vi "Sistema de Vacio 2.0.vi"() -> ()   [LabVIEW 2019]
uses:
  PortConfig.ctl
  <vilib>/Instr/_visa.llb/VISA Configure Serial Port (Instr).vi
panel:
  in  "System OFF":bool
  out "IG Filament Status 2":string
  out "VAC/ATM":bool caption="Boolean"
  out "TP AV/NAV":bool caption="Boolean"
  out "BP AV/NAV":bool caption="Boolean"
  in  "Ion Gauge":bool
  out "IG AV/NAV 2":bool caption="Boolean"
  in  "Turbo Pump":bool
  in  "System ON":bool
  in  "Backing Pump":bool
  in  "Disconnect":bool
  out "IG AV/NAV":bool caption="Boolean"
  out "Ion Gauge Controller":errorcluster
  out "Vacuum Controller":errorcluster
  out "Branking":bool
  out "Stopped":bool
  out "Starting Delay":bool
  out "Accelerating":bool
  out "Stopping Normal Delay":bool
  out "Fault Branking":bool
  out "Stopping Short Delay":bool
  out "Running":bool
  out "Backing Pump":bool
  out "Turbo Normal Speed":bool
  out "Turbo Power [W]":dbl(knob) scale=0.0..110.0
  out "Turbo Power [W]":dbl
  out "Turbo Speed":dbl(knob) scale=0.0..100.0
  out "Turbo Speed":dbl
  out "Vent Valve":bool
  out "PS Temp":dbl
  out "Internal Temp":dbl
  out "Apagado":bool
  out "B_Online":bool caption="Boolean"
  out "IG_Online":bool caption="Boolean"
  out "IG [TORR]":string
  out "IG3":dbl(knob) scale=1e-09..1e-07 scale format="%#_3e"
  out "IG":dbl(knob) scale=1e-09..0.001 scale format="%#_6e"
  out "IG1":dbl(knob) scale=1e-05..0.001 scale format="%#_3e"
  out "IG2":dbl(knob) scale=1e-07..1e-05 scale format="%#_3e"
  out "CG2 [TORR]":string
  out "CG2L":dbl(knob) scale=0.01..800.0
  out "CG2":dbl(knob) scale=0.0..800.0
  out "CG1 [TORR]":string
  out "CG1L":dbl(knob) scale=0.01..800.0
  out "CG1":dbl(knob) scale=0.0..800.0
  out "IG Filament Status":string
  out "Activo":bool
  out "ActivoIG":bool caption="Activo"
  out "Emission Current Status":string
  out "IG Code\nIG code":string
  out "IG Status":string
  out "Software Version":string
  out "Serial Number ; PIC Version":string
  out "Software Version":string
  out "TIC Model":string
  in  "Ion Gauge":refnum<visa-resource-name>="COM12"
  in  "Bombas":refnum<visa-resource-name>="COM16"
  in  "?":bool
  in  "Error In":errorcluster
  # "CONTROLS CONNECTION"
  # "VACUUM SYSTEM CONTROL"
  # "Error Handling"
  # "IG CONTROL"
  # "CONTROLLER"
  # "TURBO-PUMP DATA"
  # "TURBO-PUMP STATUS"
  # "PUMP STATUS"
  # "CONTROLLER"
  # "CONVECTRON DATA"
  # "ION GAUGE DATA"
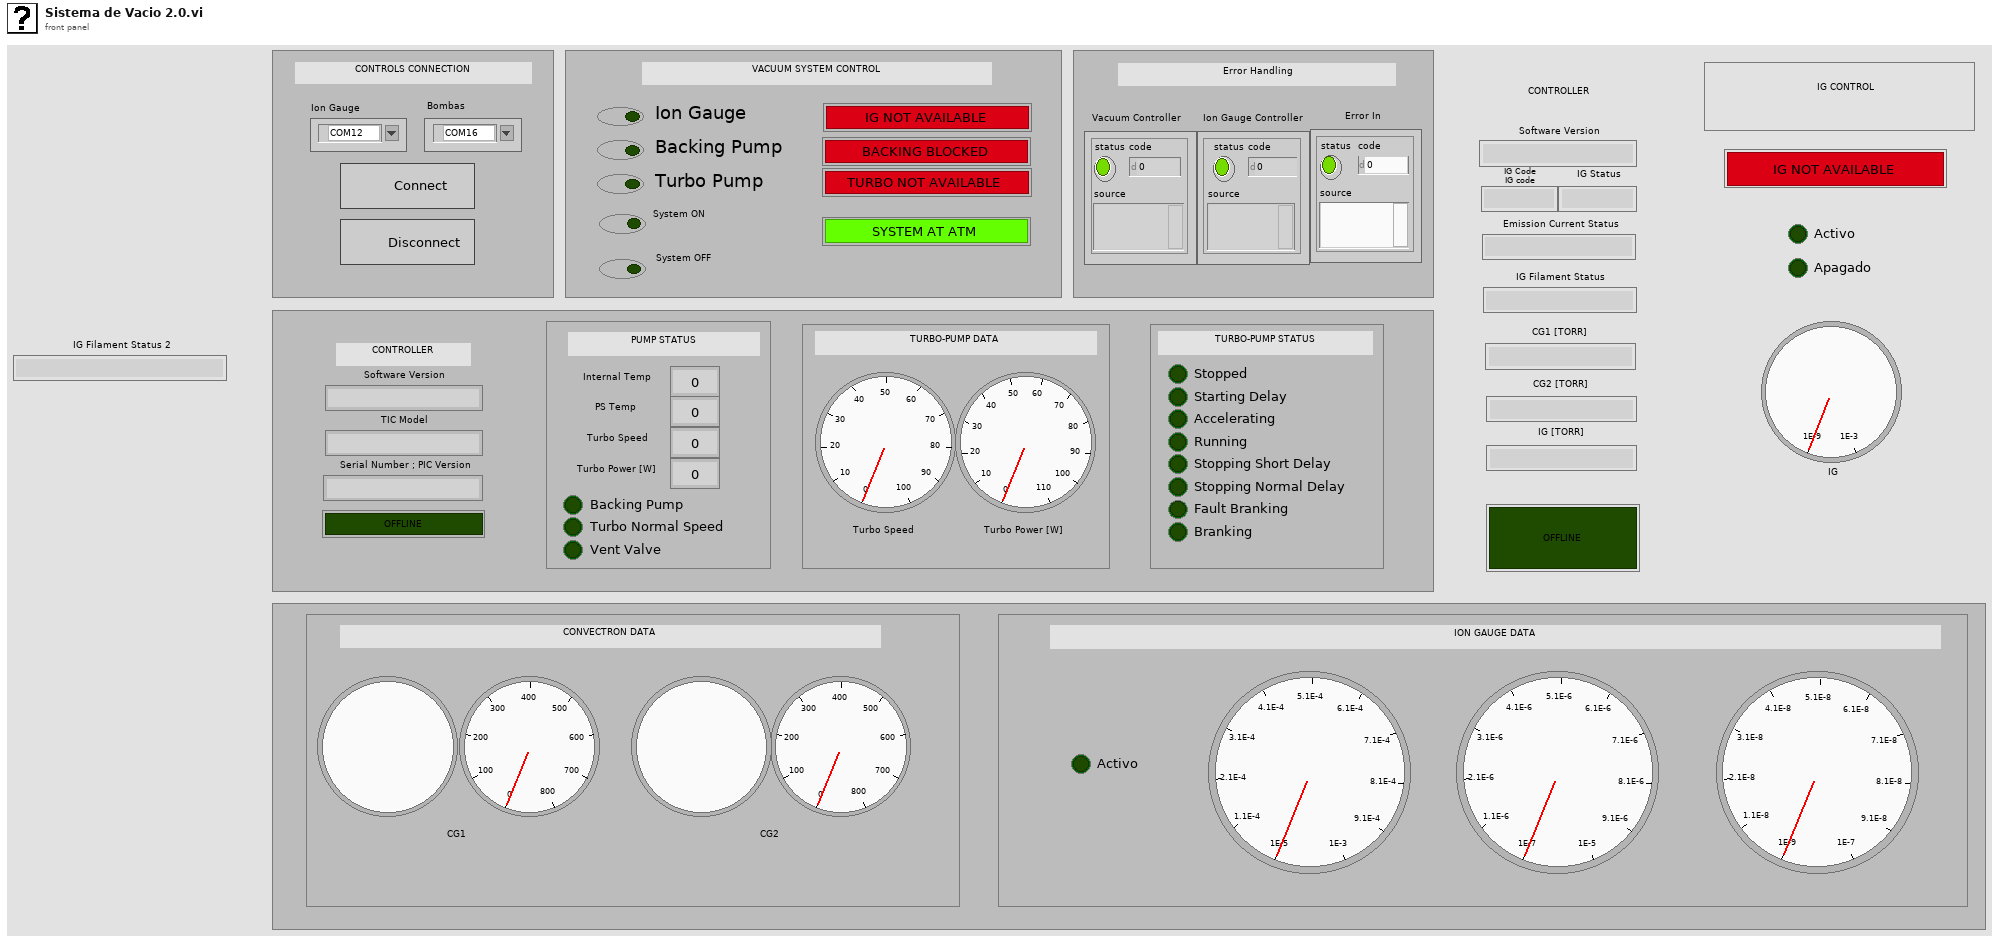
[diagram p1: front panel]
types:
  T1 = typedef "PortConfig.ctl" = cluster{"baud rate":u32, "data bits":u16, "parity":enum16{"None", "Odd", "Even", "Mark", "Space"}, "stop bits":u16}
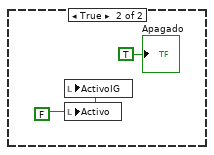
[diagram p2: hidden frame]
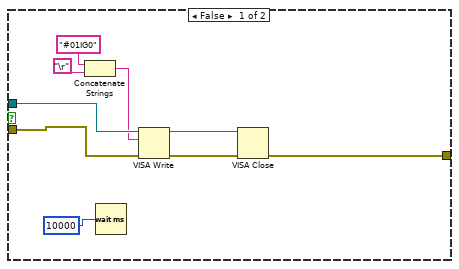
[diagram p3: hidden frame]
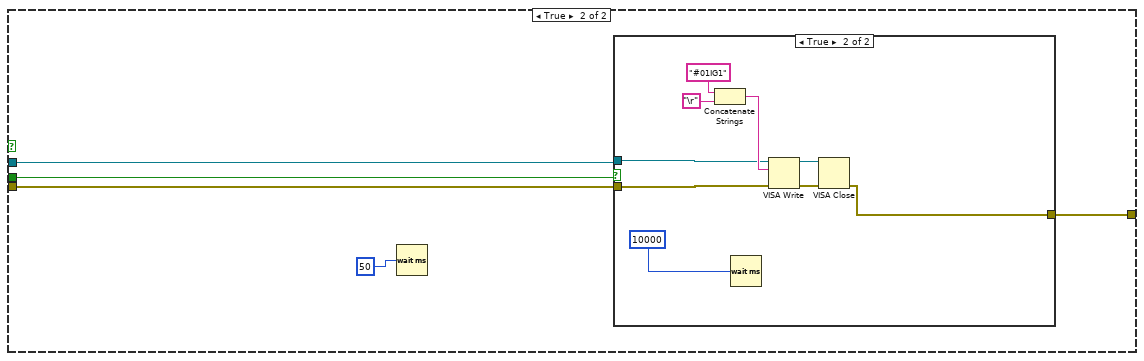
[diagram p4: hidden frame]
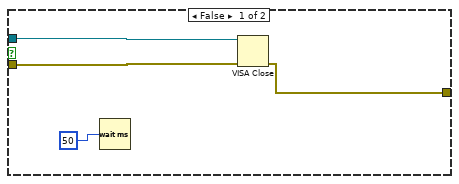
[diagram p5: hidden frame]
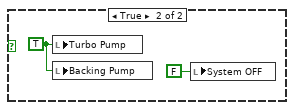
[diagram p7: hidden frame]
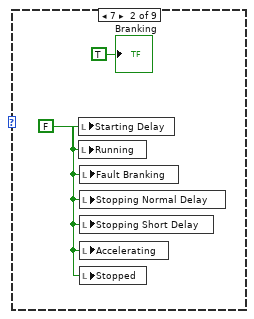
[diagram p11: hidden frame]
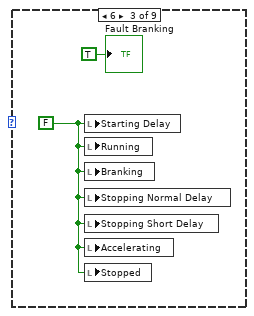
[diagram p12: hidden frame]
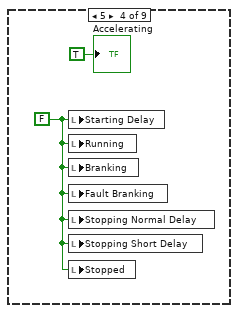
[diagram p13: hidden frame]
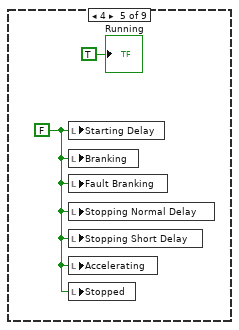
[diagram p14: hidden frame]
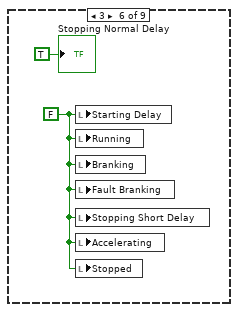
[diagram p15: hidden frame]
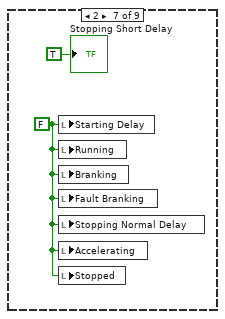
[diagram p16: hidden frame]
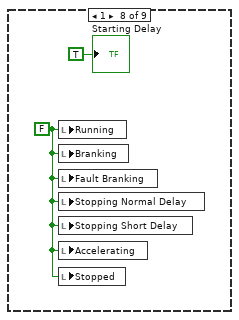
[diagram p17: hidden frame]
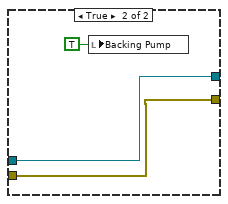
[diagram p19: hidden frame]
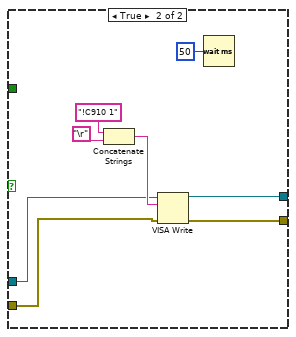
[diagram p20: hidden frame]
diagram:
  n1 = while {
    tunnel: "Error In" -> [w33]
    tunnel: [w33] -> w21
    stop <- "?" stop-if-true
    w22 = FALSE ("IG AV/NAV 2")
    w23 = " " ("CG1 [TORR]")
    w24 = 0.0 ("IG2")
    w25 = FALSE ("Apagado")
    w26 = FALSE ("Turbo Pump")
    w27 = FALSE ("Running")
    w29 = 0.0 ("Turbo Speed")
    w28 = FALSE ("IG_Online")
    w30 = " " ("TIC Model")
    n2 = local write "TP AV/NAV"(w27) -> ()
    n3 = local write "BP AV/NAV"(w27) -> ()
    n4 = local write "Running"(w27) -> ()
    n5 = local write "Branking"(w27) -> ()
    n6 = local write "Fault Branking"(w27) -> ()
    n7 = local write "Accelerating"(w27) -> ()
    n8 = local write "Stopping Normal Delay"(w27) -> ()
    n9 = local write "Stopping Short Delay"(w27) -> ()
    n10 = local write "Starting Delay"(w27) -> ()
    n11 = local write "Stopped"(w27) -> ()
    n12 = local write "VAC/ATM"(w27) -> ()
    n13 = local write "IG AV/NAV 2"(w27) -> ()
    n14 = local write "IG2"(w24) -> ()
    n15 = local write "IG1"(w24) -> ()
    n16 = local write "IG"(w24) -> ()
    n17 = local write "CG1"(w24) -> ()
    n18 = local write "CG1L"(w24) -> ()
    n19 = local write "IG3"(w24) -> ()
    n20 = local write "Apagado"(w25) -> ()
    n21 = local write "IG_Online"(w25) -> ()
    n22 = local write "ActivoIG"(w25) -> ()
    n23 = local write "Activo"(w25) -> ()
    n24 = local write "System ON"(w26) -> ()
    n25 = local write "Turbo Pump"(w26) -> ()
    n26 = local write "Backing Pump"(w26) -> ()
    n27 = local write "Ion Gauge"(w26) -> ()
    n28 = local write "IG AV/NAV 2"(w22) -> ()
    n29 = local write "IG AV/NAV"(w22) -> ()
    n30 = local write "System OFF"(w22) -> ()
    n31 = local write "CG1 [TORR]"(w23) -> ()
    n32 = local write "CG2 [TORR]"(w23) -> ()
    n33 = local write "IG [TORR]"(w23) -> ()
    n34 = local write "IG Filament Status"(w23) -> ()
    n35 = local write "Emission Current Status"(w23) -> ()
    n36 = local write "Software Version"(w23) -> ()
    n37 = local write "IG Code\nIG code"(w23) -> ()
    n38 = local write "IG Status"(w23) -> ()
    n39 = local write "Turbo Speed"(w29) -> ()
    n40 = local write "Turbo Speed"(w29) -> ()
    n41 = local write "Turbo Power [W]"(w29) -> ()
    n42 = local write "Turbo Power [W]"(w29) -> ()
    n43 = local write "Internal Temp"(w29) -> ()
    n44 = local write "PS Temp"(w29) -> ()
    n45 = local write "TIC Model"(w30) -> ()
    n46 = local write "Software Version"(w30) -> ()
    n47 = local write "Serial Number ; PIC Version"(w30) -> ()
    n48 = local write "IG_Online"(w28) -> ()
    n49 = local write "B_Online"(w28) -> ()
    n50 = local write "Vent Valve"(w28) -> ()
    n51 = local write "Turbo Normal Speed"(w28) -> ()
    n52 = local write "Backing Pump"(w28) -> ()
    n53 = Wait (ms)(milliseconds to wait=u32 200) -> ()  [unwired: 1 out]
  }
  n54 = flat-sequence {
    tunnel: w21 -> [w52]
    tunnel: [w52] -> w14
    tunnel: [w37] -> w13
    tunnel: [w36] -> w12
    tunnel: [w35] -> w11
    tunnel: [w34] -> w10
    tunnel: [w113] -> w9
    tunnel: w14 -> [w113]
    tunnel: w13 -> [w98]
    tunnel: w12 -> [w97]
    tunnel: w11 -> [w80]
    tunnel: w10 -> [w79]
    tunnel: [w78] -> w8
    tunnel: [w77] -> w7
    tunnel: [w59] -> w6
    tunnel: [w58] -> w5
    tunnel: [w53] -> w2
    tunnel: [w55] -> w1
    tunnel: [w120] -> w15
    tunnel: [w121] -> w16
    tunnel: [w122] -> w17
    tunnel: [w123] -> w18
    tunnel: [w124] -> w19
    tunnel: w9 -> [w124]
    tunnel: w8 -> [w119]
    tunnel: w7 -> [w118]
    tunnel: w6 -> [w117]
    tunnel: w5 -> [w116]
    tunnel: [w114] -> w4
    tunnel: [w115] -> w3
    tunnel: w2 -> [w115]
    tunnel: w1 -> [w114]
    frame #0 {
      n55 = Unbundle By Name(T1 {"baud rate"=9600, "data bits"=8, "parity"=enum."None", "stop bits"=10} ("Serial Settings")) -> ("data bits"=w48:u16, "parity"=w47:enum16{"None", "Odd", "Even", "Mark", "Space"}, "stop bits"=w49:u16)  [unwired: 1 out]
      n56 = Unbundle By Name(T1 {"baud rate"=9600, "data bits"=8, "parity"=enum."None", "stop bits"=10} ("Serial Settings")) -> ("data bits"=w43:u16, "parity"=w42:enum16{"None", "Odd", "Even", "Mark", "Space"}, "stop bits"=w44:u16)  [unwired: 1 out]
      n57 = call-poly "VISA Configure Serial Port"("VISA resource name"="Bombas", "data bits (8)"=w48, "parity (0:none)"=w47, "stop bits (10: 1 bit)"=w49) -> ("VISA resource name out"=w39:refnum<visa-resource-name>, "error out"=w38:errorcluster)  [unwired: 10 in]
      n58 = call-poly "VISA Configure Serial Port"("VISA resource name"="Ion Gauge", "data bits (8)"=w43, "parity (0:none)"=w42, "stop bits (10: 1 bit)"=w44) -> ("VISA resource name out"=w41:refnum<visa-resource-name>, "error out"=w40:errorcluster)  [unwired: 10 in]
      n59 = VISA Flush I/O Buffer(VISA resource name=w39, error in (no error)=w38) -> (VISA resource name out=w37:refnum<visa-resource-name>, error out=w36:errorcluster)  [unwired: 1 in]
      n60 = VISA Flush I/O Buffer(VISA resource name=w41, error in (no error)=w40) -> (VISA resource name out=w35:refnum<visa-resource-name>, error out=w34:errorcluster)  [unwired: 1 in]
    }
    frame #1 {
      n61 = Concatenate Strings("?V910", "\r") -> (w110:string)
      n62 = Concatenate Strings("#01IGS", "\r") -> (w90:string)
      n63 = VISA Write(VISA resource name=w98, write buffer=w110, error in (no error)=w97) -> (VISA resource name out=w109:refnum<visa-resource-name>, error out=w108:errorcluster)  [unwired: 1 out]
      n64 = VISA Write(VISA resource name=w80, write buffer=w90, error in (no error)=w79) -> (VISA resource name out=w94:refnum<visa-resource-name>, error out=w95:errorcluster)  [unwired: 1 out]
      n65 = VISA Read(VISA resource name=w109, byte count=u32 10, error in (no error)=w108) -> (VISA resource name out=w100:refnum<visa-resource-name>, read buffer=w105:string, error out=w99:errorcluster)  [unwired: 1 out]
      n66 = VISA Read(VISA resource name=w94, byte count=13, error in (no error)=w95) -> (VISA resource name out=w78:refnum<visa-resource-name>, read buffer=w96:string, error out=w77:errorcluster)  [unwired: 1 out]
      n67 = Search/Split String(string=w105, search string/char (-)=" ") -> (match + rest of string=w103:string)  [unwired: 1 in, 2 out]
      n68 = Search/Split String(string=w96, search string/char (-)="IG ", offset (0)=3) -> (match + rest of string=w81:string)  [unwired: 2 out]
      "IG Filament Status 2" <- w81
      n69 = Search/Split String(string=w103, search string/char (-)=";") -> (substring before match=w102:string)  [unwired: 1 in, 2 out]
      n70 = Equal?(x=" 0", y=w102) -> (x = y?=w54:bool)
      n71 = Not(x=w54) -> (.not. x?=w53:bool)
      n72 = Search/Split String(string=w81, search string/char (-)="O", offset (0)=3) -> (match + rest of string=w82:string)  [unwired: 2 out]
      n73 = VISA Flush I/O Buffer(VISA resource name=w100, error in (no error)=w99) -> (VISA resource name out=w61:refnum<visa-resource-name>, error out=w60:errorcluster)  [unwired: 1 in]
      n74 = local write "Backing Pump"(w53) -> ()
      n75 = Concatenate Strings("?V907", "\r") -> (w71:string)
      n76 = Concatenate Strings("OFF", "\r") -> (w83:string)
      n77 = VISA Write(VISA resource name=w61, write buffer=w71, error in (no error)=w60) -> (VISA resource name out=w70:refnum<visa-resource-name>, error out=w69:errorcluster)  [unwired: 1 out]
      n78 = Equal?(x=w83, y=w82) -> (x = y?=w57:bool)
      n79 = Not(x=w57) -> (.not. x?=w56:bool)
      n80 = VISA Read(VISA resource name=w70, byte count=u32 10, error in (no error)=w69) -> (VISA resource name out=w75:refnum<visa-resource-name>, read buffer=w66:string, error out=w76:errorcluster)  [unwired: 1 out]
      n81 = local write "Ion Gauge"(w56) -> ()
      n82 = Search/Split String(string=w66, search string/char (-)=" ") -> (match + rest of string=w64:string)  [unwired: 1 in, 2 out]
      n83 = VISA Flush I/O Buffer(VISA resource name=w75, error in (no error)=w76) -> (VISA resource name out=w59:refnum<visa-resource-name>, error out=w58:errorcluster)  [unwired: 1 in]
      n84 = Search/Split String(string=w64, search string/char (-)=";") -> (substring before match=w63:string)  [unwired: 1 in, 2 out]
      n85 = Equal?(x=" 0", y=w63) -> (x = y?=w74:bool)
      n86 = Not(x=w74) -> (.not. x?=w55:bool)
      n87 = local write "Turbo Pump"(w55) -> ()
    }
    frame #2 {
      n88 = VISA Flush I/O Buffer(VISA resource name=w117, error in (no error)=w116) -> (VISA resource name out=w121:refnum<visa-resource-name>, error out=w120:errorcluster)  [unwired: 1 in]
      n89 = VISA Flush I/O Buffer(VISA resource name=w119, error in (no error)=w118) -> (VISA resource name out=w123:refnum<visa-resource-name>, error out=w122:errorcluster)  [unwired: 1 in]
    }
  }
  n90 = while {
    tunnel: w19 -> [_]
    tunnel: w18 -> [w245]
    tunnel: w17 -> [w244]
    tunnel: w16 -> [w243]
    tunnel: w15 -> [w242]
    shift-right: [w138] -> _
    shift-left: w3 -> [w184]
    shift-right: [w137] -> _
    shift-left: w4 -> [w185]
    stop <- "Disconnect" stop-if-true
    n91 = flat-sequence {
      tunnel: w242 -> [w464]
      tunnel: w243 -> [w465]
      tunnel: [w465] -> w187
      tunnel: [w464] -> w186
      tunnel: w185 -> [w459]
      tunnel: w184 -> [w463]
      tunnel: [w462] -> w145
      tunnel: [w461] -> w144
      tunnel: ["Backing Pump"] -> w143
      tunnel: ["Turbo Pump"] -> w142
      tunnel: [w471] -> w240
      tunnel: [w470] -> w239
      tunnel: w187 -> [w491]
      tunnel: w186 -> [w490]
      tunnel: [w469] -> w150
      tunnel: [w468] -> w148
      tunnel: [w467] -> w147
      tunnel: [w466] -> w146
      tunnel: w145 -> [w467]
      tunnel: w144 -> [w468]
      tunnel: w143 -> [w466]
      tunnel: w142 -> [w469]
      tunnel: w240 -> [w506]
      tunnel: w239 -> [w512]
      tunnel: [w503] -> w238
      tunnel: [w502] -> w237
      tunnel: [w500] -> w157
      tunnel: [w499] -> w154
      tunnel: [w498] -> w151
      tunnel: w150 -> [w497]
      tunnel: [w497] -> w149
      tunnel: w148 -> [w498]
      tunnel: w147 -> [w500]
      tunnel: w146 -> [w499]
      tunnel: w238 -> [w527]
      tunnel: w237 -> [w526]
      tunnel: [w523] -> w236
      tunnel: [w522] -> w235
      tunnel: [w521] -> w163
      tunnel: [w520] -> w158
      tunnel: w157 -> [w519]
      tunnel: [w519] -> w156
      tunnel: w154 -> [w518]
      tunnel: [w518] -> w153
      tunnel: w151 -> [w521]
      tunnel: w149 -> [w520]
      tunnel: w236 -> [w554]
      tunnel: w235 -> [w553]
      tunnel: [w546] -> w234
      tunnel: [w545] -> w233
      tunnel: w163 -> [w542]
      tunnel: [w542] -> w162
      tunnel: [w541] -> w160
      tunnel: w158 -> [w541]
      tunnel: w156 -> [w540]
      tunnel: [w540] -> w155
      tunnel: w153 -> [w539]
      tunnel: [w539] -> w152
      tunnel: w234 -> [w578]
      tunnel: w233 -> [w577]
      tunnel: [w570] -> w232
      tunnel: [w569] -> w231
      tunnel: [w565] -> w169
      tunnel: [w564] -> w166
      tunnel: w162 -> [w563]
      tunnel: [w563] -> w161
      tunnel: w160 -> [w562]
      tunnel: [w562] -> w159
      tunnel: w155 -> [w565]
      tunnel: w152 -> [w564]
      tunnel: [w561] -> w135
      tunnel: w232 -> [w594]
      tunnel: w231 -> [w593]
      tunnel: [w592] -> w230
      tunnel: [w591] -> w229
      tunnel: [w590] -> w175
      tunnel: [w589] -> w172
      tunnel: w169 -> [w588]
      tunnel: [w588] -> w168
      tunnel: w166 -> [w587]
      tunnel: [w587] -> w165
      tunnel: w161 -> [w590]
      tunnel: w159 -> [w589]
      tunnel: [w586] -> w136
      tunnel: w135 -> [w586]
      tunnel: [w585] -> w131
      tunnel: w130 -> [w585]
      tunnel: w230 -> [w621]
      tunnel: w229 -> [w620]
      tunnel: [w616] -> w228
      tunnel: [w615] -> w227
      tunnel: w175 -> [w613]
      tunnel: [w613] -> w174
      tunnel: w172 -> [w612]
      tunnel: [w612] -> w171
      tunnel: w168 -> [w611]
      tunnel: [w611] -> w167
      tunnel: w165 -> [w610]
      tunnel: [w610] -> w164
      tunnel: w136 -> [w609]
      tunnel: [w609] -> w133
      tunnel: w131 -> [w608]
      tunnel: [w608] -> w128
      tunnel: w228 -> [w646]
      tunnel: w227 -> [w645]
      tunnel: [w642] -> w226
      tunnel: [w641] -> w225
      tunnel: [w639] -> w183
      tunnel: [w638] -> w181
      tunnel: w174 -> [w637]
      tunnel: [w637] -> w173
      tunnel: w171 -> [w636]
      tunnel: [w636] -> w170
      tunnel: w167 -> [w639]
      tunnel: w164 -> [w638]
      tunnel: [w635] -> w134
      tunnel: w133 -> [w635]
      tunnel: [w634] -> w129
      tunnel: w128 -> [w634]
      tunnel: w226 -> [w674]
      tunnel: w225 -> [w673]
      tunnel: [w667] -> w193
      tunnel: [w666] -> w192
      tunnel: w183 -> [w665]
      tunnel: [w665] -> w182
      tunnel: w181 -> [w664]
      tunnel: [w664] -> w180
      tunnel: [w663] -> w179
      tunnel: [w662] -> w177
      tunnel: w173 -> [w663]
      tunnel: w170 -> [w662]
      tunnel: w134 -> [w661]
      tunnel: [w661] -> w132
      tunnel: w129 -> [w660]
      tunnel: [w660] -> w126
      tunnel: w193 -> [w711]
      tunnel: w192 -> [w710]
      tunnel: [w709] -> w191
      tunnel: [w708] -> w189
      tunnel: w182 -> [w707]
      tunnel: w180 -> [w704]
      tunnel: w179 -> [w706]
      tunnel: [w706] -> w178
      tunnel: w177 -> [w705]
      tunnel: [w705] -> w176
      tunnel: [w704] -> w140
      tunnel: w132 -> [w703]
      tunnel: [w701] -> w127
      tunnel: w126 -> [w701]
      tunnel: w191 -> [w751]
      tunnel: [w749] -> w190
      tunnel: w189 -> [w750]
      tunnel: [w748] -> w188
      tunnel: w178 -> [w747]
      tunnel: w176 -> [w745]
      tunnel: [w746] -> w141
      tunnel: w140 -> [w746]
      tunnel: [w745] -> w139
      tunnel: w127 -> [w744]
      tunnel: w190 -> [w786]
      tunnel: w188 -> [w787]
      tunnel: [w789] -> w138
      tunnel: w141 -> [w789]
      tunnel: [w788] -> w137
      tunnel: w139 -> [w788]
      frame #0 {
        n92 = Not Equal?(x="Backing Pump", y=w463) -> (x != y?=w462:bool)
        n93 = Not Equal?(x="Turbo Pump", y=w459) -> (x != y?=w461:bool)
      }
      frame #1 {
        n94 = Concatenate Strings("?S902", "\r") -> (w494:string)
        n95 = VISA Write(VISA resource name=w491, write buffer=w494, error in (no error)=w490) -> (VISA resource name out=w495:refnum<visa-resource-name>, error out=w496:errorcluster)  [unwired: 1 out]
        n96 = VISA Read(VISA resource name=w495, byte count=u32 38, error in (no error)=w496) -> (VISA resource name out=w471:refnum<visa-resource-name>, read buffer=w475:string, error out=w470:errorcluster)  [unwired: 1 out]
        n97 = Search/Split String(string=w475, search string/char (-)=" ") -> (match + rest of string=w486:string)  [unwired: 1 in, 2 out]
        n98 = Search/Split String(string=w486, search string/char (-)=";") -> (substring before match=w474:string, match + rest of string=w485:string)  [unwired: 1 in, 1 out]
        "TIC Model" <- w474
        n99 = Search/Split String(string=w485, search string/char (-)=";0") -> (substring before match=w480:string, match + rest of string=w476:string)  [unwired: 1 in, 1 out]
        n100 = Search and Replace String(input string=w480, search string=";", replace string="" ("replace string (\"\")")) -> (result string=→"Software Version":string)  [unwired: 5 in, 3 out]
        n101 = Search and Replace String(input string=w476, search string=";", replace string="" ("replace string (\"\")")) -> (result string=→"Serial Number ; PIC Version":string)  [unwired: 5 in, 3 out]
        n102 = Equal?(x=w474, y=" TIC100") -> (x = y?=→"B_Online":bool)
      }
      frame #2 {
        n103 = Concatenate Strings("?V919", "\r") -> (w515:string)
        n104 = VISA Write(VISA resource name=w506, write buffer=w515, error in (no error)=w512) -> (VISA resource name out=w514:refnum<visa-resource-name>, error out=w513:errorcluster)  [unwired: 1 out]
        n105 = VISA Read(VISA resource name=w514, byte count=u32 16, error in (no error)=w513) -> (VISA resource name out=w503:refnum<visa-resource-name>, read buffer=w501:string, error out=w502:errorcluster)  [unwired: 1 out]
        n106 = Search/Split String(string=w501, search string/char (-)=" ") -> (match + rest of string=w504:string)  [unwired: 1 in, 2 out]
        n107 = Fract/Exp String To Number(use system decimal point (T)=TRUE, string=w504) -> (number=w509:dbl)  [unwired: 2 in, 1 out]
        n108 = Subtract(x=w509, y=274.0 ("x")) -> (x-y=→"Internal Temp":dbl)
      }
      frame #3 {
        n109 = Concatenate Strings("?V920", "\r") -> (w536:string)
        n110 = VISA Write(VISA resource name=w527, write buffer=w536, error in (no error)=w526) -> (VISA resource name out=w535:refnum<visa-resource-name>, error out=w534:errorcluster)  [unwired: 1 out]
        n111 = VISA Read(VISA resource name=w535, byte count=u32 16, error in (no error)=w534) -> (VISA resource name out=w523:refnum<visa-resource-name>, read buffer=w524:string, error out=w522:errorcluster)  [unwired: 1 out]
        n112 = Search/Split String(string=w524, search string/char (-)=" ") -> (match + rest of string=w528:string)  [unwired: 1 in, 2 out]
        n113 = Fract/Exp String To Number(use system decimal point (T)=TRUE, string=w528) -> (number=w531:dbl)  [unwired: 2 in, 1 out]
        n114 = Subtract(x=w531, y=274.0 ("x")) -> (x-y=→"PS Temp":dbl)
      }
      frame #4 {
        n115 = Concatenate Strings("?V922", "\r") -> (w558:string)
        n116 = VISA Write(VISA resource name=w554, write buffer=w558, error in (no error)=w553) -> (VISA resource name out=w557:refnum<visa-resource-name>, error out=w556:errorcluster)  [unwired: 1 out]
        n117 = VISA Read(VISA resource name=w557, byte count=u32 13, error in (no error)=w556) -> (VISA resource name out=w546:refnum<visa-resource-name>, read buffer=w551:string, error out=w545:errorcluster)  [unwired: 1 out]
        n118 = Search/Split String(string=w551, search string/char (-)=" ") -> (match + rest of string=w549:string)  [unwired: 1 in, 2 out]
        n119 = Search/Split String(string=w549, search string/char (-)=";") -> (substring before match=w548:string)  [unwired: 1 in, 2 out]
        n120 = Equal?(x=" 0", y=w548) -> (x = y?=w544:bool)
        n121 = Not(x=w544) -> (.not. x?=→"Vent Valve":bool)
      }
      frame #5 {
        n122 = Concatenate Strings("?V905", "\r") -> (w582:string)
        n123 = VISA Write(VISA resource name=w578, write buffer=w582, error in (no error)=w577) -> (VISA resource name out=w581:refnum<visa-resource-name>, error out=w580:errorcluster)  [unwired: 1 out]
        n124 = VISA Read(VISA resource name=w581, byte count=u32 13, error in (no error)=w580) -> (VISA resource name out=w570:refnum<visa-resource-name>, read buffer=w573:string, error out=w569:errorcluster)  [unwired: 1 out]
        n125 = Search/Split String(string=w573, search string/char (-)=" ") -> (match + rest of string=w575:string)  [unwired: 1 in, 2 out]
        n126 = Search/Split String(string=w575, search string/char (-)=";") -> (substring before match=w572:string)  [unwired: 1 in, 2 out]
        n127 = Fract/Exp String To Number(use system decimal point (T)=TRUE, string=w572) -> (number=w567:dbl)  [unwired: 2 in, 1 out]
        "Turbo Speed" <- w567
        "Turbo Speed" <- w567
        n128 = Greater Or Equal?(x=w567, y=4.0) -> (x >= y?=w568:bool)
        n129 = Not(x=w568) -> (.not. x?=w561:bool)
        "BP AV/NAV" <- w561
      }
      frame #6 {
        n130 = Concatenate Strings("?V906", "\r") -> (w605:string)
        n131 = VISA Write(VISA resource name=w594, write buffer=w605, error in (no error)=w593) -> (VISA resource name out=w604:refnum<visa-resource-name>, error out=w603:errorcluster)  [unwired: 1 out]
        n132 = VISA Read(VISA resource name=w604, byte count=u32 13, error in (no error)=w603) -> (VISA resource name out=w592:refnum<visa-resource-name>, read buffer=w598:string, error out=w591:errorcluster)  [unwired: 1 out]
        n133 = Search/Split String(string=w598, search string/char (-)=" ") -> (match + rest of string=w600:string)  [unwired: 1 in, 2 out]
        n134 = Search/Split String(string=w600, search string/char (-)=";") -> (substring before match=w597:string)  [unwired: 1 in, 2 out]
        n135 = Fract/Exp String To Number(use system decimal point (T)=TRUE, string=w597) -> (number=→"Turbo Power [W]" →"Turbo Power [W]":dbl)  [unwired: 2 in, 1 out]
      }
      frame #7 {
        n136 = Concatenate Strings("?V907", "\r") -> (w624:string)
        n137 = VISA Write(VISA resource name=w621, write buffer=w624, error in (no error)=w620) -> (VISA resource name out=w625:refnum<visa-resource-name>, error out=w626:errorcluster)  [unwired: 1 out]
        n138 = VISA Read(VISA resource name=w625, byte count=u32 10, error in (no error)=w626) -> (VISA resource name out=w618:refnum<visa-resource-name>, read buffer=w629:string, error out=w617:errorcluster)  [unwired: 1 out]
        n139 = Search/Split String(string=w629, search string/char (-)=" ") -> (match + rest of string=w631:string)  [unwired: 1 in, 2 out]
        n140 = VISA Flush I/O Buffer(VISA resource name=w618, error in (no error)=w617) -> (VISA resource name out=w616:refnum<visa-resource-name>, error out=w615:errorcluster)  [unwired: 1 in]
        n141 = Search/Split String(string=w631, search string/char (-)=";") -> (substring before match=w632:string)  [unwired: 1 in, 2 out]
        n142 = Equal?(x=" 0", y=w632) -> (x = y?=w619:bool)
        n143 = Not(x=w619) -> (.not. x?=→"Turbo Normal Speed":bool)
      }
      frame #8 {
        n144 = Concatenate Strings("?V910", "\r") -> (w656:string)
        n145 = VISA Write(VISA resource name=w646, write buffer=w656, error in (no error)=w645) -> (VISA resource name out=w655:refnum<visa-resource-name>, error out=w654:errorcluster)  [unwired: 1 out]
        n146 = VISA Read(VISA resource name=w655, byte count=u32 10, error in (no error)=w654) -> (VISA resource name out=w644:refnum<visa-resource-name>, read buffer=w651:string, error out=w643:errorcluster)  [unwired: 1 out]
        n147 = Search/Split String(string=w651, search string/char (-)=" ") -> (match + rest of string=w649:string)  [unwired: 1 in, 2 out]
        n148 = Search/Split String(string=w649, search string/char (-)=";") -> (substring before match=w648:string)  [unwired: 1 in, 2 out]
        n149 = Equal?(x=" 0", y=w648) -> (x = y?=w659:bool)
        n150 = Not(x=w659) -> (.not. x?=→"Backing Pump":bool)
        n151 = VISA Flush I/O Buffer(VISA resource name=w644, error in (no error)=w643) -> (VISA resource name out=w642:refnum<visa-resource-name>, error out=w641:errorcluster)  [unwired: 1 in]
      }
      frame #9 {
        n152 = Concatenate Strings("?V904", "\r") -> (w677:string)
        n153 = VISA Write(VISA resource name=w674, write buffer=w677, error in (no error)=w673) -> (VISA resource name out=w678:refnum<visa-resource-name>, error out=w679:errorcluster)  [unwired: 1 out]
        n154 = VISA Read(VISA resource name=w678, byte count=u32 10, error in (no error)=w679) -> (VISA resource name out=w672:refnum<visa-resource-name>, read buffer=w682:string, error out=w671:errorcluster)  [unwired: 1 out]
        n155 = Search/Split String(string=w682, search string/char (-)=" ") -> (match + rest of string=w684:string)  [unwired: 1 in, 2 out]
        n156 = Search/Split String(string=w684, search string/char (-)=";") -> (substring before match=w669:string)  [unwired: 1 in, 2 out]
        n157 = Fract/Exp String To Number(use system decimal point (T)=FALSE, string=w669) -> (number=w668:dbl)  [unwired: 2 in, 1 out]
        n158 = case shown="0" w668 {
          frame 8, Default {
          }
          frame 7 {
            w685 = FALSE ("Starting Delay")
            n159 = local write "Starting Delay"(w685) -> ()
            n160 = local write "Running"(w685) -> ()
            n161 = local write "Fault Branking"(w685) -> ()
            n162 = local write "Stopping Normal Delay"(w685) -> ()
            n163 = local write "Stopping Short Delay"(w685) -> ()
            n164 = local write "Accelerating"(w685) -> ()
            n165 = local write "Stopped"(w685) -> ()
            "Branking" <- TRUE ("Branking")
          }
          frame 6 {
            w687 = FALSE ("Starting Delay")
            n166 = local write "Starting Delay"(w687) -> ()
            n167 = local write "Running"(w687) -> ()
            n168 = local write "Branking"(w687) -> ()
            n169 = local write "Stopping Normal Delay"(w687) -> ()
            n170 = local write "Stopping Short Delay"(w687) -> ()
            n171 = local write "Accelerating"(w687) -> ()
            n172 = local write "Stopped"(w687) -> ()
            "Fault Branking" <- TRUE ("Fault Branking")
          }
          frame 5 {
            w689 = FALSE ("Starting Delay")
            n173 = local write "Starting Delay"(w689) -> ()
            n174 = local write "Running"(w689) -> ()
            n175 = local write "Branking"(w689) -> ()
            n176 = local write "Fault Branking"(w689) -> ()
            n177 = local write "Stopping Normal Delay"(w689) -> ()
            n178 = local write "Stopping Short Delay"(w689) -> ()
            n179 = local write "Stopped"(w689) -> ()
            "Accelerating" <- TRUE ("Accelerating")
          }
          frame 4 {
            w691 = FALSE ("Starting Delay")
            n180 = local write "Starting Delay"(w691) -> ()
            n181 = local write "Branking"(w691) -> ()
            n182 = local write "Fault Branking"(w691) -> ()
            n183 = local write "Stopping Normal Delay"(w691) -> ()
            n184 = local write "Stopping Short Delay"(w691) -> ()
            n185 = local write "Accelerating"(w691) -> ()
            n186 = local write "Stopped"(w691) -> ()
            "Running" <- TRUE ("Running")
          }
          frame 3 {
            w694 = FALSE ("Starting Delay")
            n187 = local write "Starting Delay"(w694) -> ()
            n188 = local write "Running"(w694) -> ()
            n189 = local write "Branking"(w694) -> ()
            n190 = local write "Fault Branking"(w694) -> ()
            n191 = local write "Stopping Short Delay"(w694) -> ()
            n192 = local write "Accelerating"(w694) -> ()
            n193 = local write "Stopped"(w694) -> ()
            "Stopping Normal Delay" <- TRUE ("Stopping Normal Delay")
          }
          frame 2 {
            w695 = FALSE ("Starting Delay")
            n194 = local write "Starting Delay"(w695) -> ()
            n195 = local write "Running"(w695) -> ()
            n196 = local write "Branking"(w695) -> ()
            n197 = local write "Fault Branking"(w695) -> ()
            n198 = local write "Stopping Normal Delay"(w695) -> ()
            n199 = local write "Accelerating"(w695) -> ()
            n200 = local write "Stopped"(w695) -> ()
            "Stopping Short Delay" <- TRUE ("Stopping Short Delay")
          }
          frame 1 {
            w697 = FALSE ("Running")
            n201 = local write "Running"(w697) -> ()
            n202 = local write "Branking"(w697) -> ()
            n203 = local write "Fault Branking"(w697) -> ()
            n204 = local write "Stopping Normal Delay"(w697) -> ()
            n205 = local write "Stopping Short Delay"(w697) -> ()
            n206 = local write "Accelerating"(w697) -> ()
            n207 = local write "Stopped"(w697) -> ()
            "Starting Delay" <- TRUE ("Starting Delay")
          }
          frame 0 {
            w700 = FALSE ("Starting Delay")
            n208 = local write "Starting Delay"(w700) -> ()
            n209 = local write "Running"(w700) -> ()
            n210 = local write "Branking"(w700) -> ()
            n211 = local write "Fault Branking"(w700) -> ()
            n212 = local write "Stopping Normal Delay"(w700) -> ()
            n213 = local write "Stopping Short Delay"(w700) -> ()
            n214 = local write "Accelerating"(w700) -> ()
            "Stopped" <- TRUE ("Stopped")
          }
        }
        n215 = VISA Flush I/O Buffer(VISA resource name=w672, error in (no error)=w671) -> (VISA resource name out=w667:refnum<visa-resource-name>, error out=w666:errorcluster)  [unwired: 1 in]
      }
      frame #10 {
        n216 = Not(x=w703) -> (.not. x?=w702:bool)
        n217 = case shown="True" w707 {
          tunnel: w711 -> [w713 w719]
          tunnel: w710 -> [w712 w718]
          tunnel: w704 -> [_ w717]
          tunnel: [w713 w715] -> w709
          tunnel: [w712 w716] -> w708
          tunnel: w702 -> [_ w714]
          frame False {
          }
          frame True {
            n218 = case shown="False" w717 {
              tunnel: w719 -> [w722 w740]
              tunnel: w718 -> [w720 w739]
              tunnel: [w723 w738] -> w715
              tunnel: [w721 w737] -> w716
              tunnel: w714 -> [w724 _]
              frame False {
                n219 = case shown="False" w724 {
                  tunnel: [w729 w734] -> w723
                  tunnel: w722 -> [w727 w734]
                  tunnel: [w728 w733] -> w721
                  tunnel: w720 -> [w726 w733]
                  frame False {
                    n220 = Concatenate Strings("!C910 0", "\r") -> (w732:string)
                    n221 = VISA Write(VISA resource name=w727, write buffer=w732, error in (no error)=w726) -> (VISA resource name out=w729:refnum<visa-resource-name>, error out=w728:errorcluster)  [unwired: 1 out]
                    n222 = Wait (ms)(milliseconds to wait=u32 50) -> ()  [unwired: 1 out]
                  }
                  frame True {
                    n223 = local write "Backing Pump"(TRUE ("Backing Pump")) -> ()
                  }
                }
              }
              frame True {
                n224 = Concatenate Strings("!C910 1", "\r") -> (w741:string)
                n225 = VISA Write(VISA resource name=w740, write buffer=w741, error in (no error)=w739) -> (VISA resource name out=w738:refnum<visa-resource-name>, error out=w737:errorcluster)  [unwired: 1 out]
                n226 = Wait (ms)(milliseconds to wait=u32 50) -> ()  [unwired: 1 out]
              }
            }
          }
        }
      }
      frame #11 {
        n227 = case shown="True" w747 {
          tunnel: [w753 w757] -> w749
          tunnel: w751 -> [w753 w759]
          tunnel: [w752 w756] -> w748
          tunnel: w750 -> [w752 w758]
          tunnel: w745 -> [_ w755]
          tunnel: w744 -> [_ w754]
          frame False {
          }
          frame True {
            n228 = case shown="True" w755 {
              tunnel: [w764 w769] -> w757
              tunnel: [w763 w768] -> w756
              tunnel: w759 -> [w762 w771]
              tunnel: w758 -> [w761 w770]
              tunnel: w754 -> [_ w772]
              frame False {
                n229 = Concatenate Strings("!C904 0", "\r") -> (w767:string)
                n230 = VISA Write(VISA resource name=w762, write buffer=w767, error in (no error)=w761) -> (VISA resource name out=w764:refnum<visa-resource-name>, error out=w763:errorcluster)  [unwired: 1 out]
                n231 = Wait (ms)(milliseconds to wait=u32 50) -> ()  [unwired: 1 out]
              }
              frame True {
                n232 = case shown="True" w772 {
                  tunnel: w771 -> [w774 w780]
                  tunnel: w770 -> [w773 w779]
                  tunnel: [w774 w778] -> w769
                  tunnel: [w773 w777] -> w768
                  frame False {
                    n233 = local write "Turbo Pump"(FALSE ("Turbo Pump")) -> ()
                  }
                  frame True {
                    n234 = Concatenate Strings("!C904 1", "\r") -> (w781:string)
                    n235 = VISA Write(VISA resource name=w780, write buffer=w781, error in (no error)=w779) -> (VISA resource name out=w778:refnum<visa-resource-name>, error out=w777:errorcluster)  [unwired: 1 out]
                    n236 = Wait (ms)(milliseconds to wait=u32 50) -> ()  [unwired: 1 out]
                  }
                }
              }
            }
          }
        }
      }
      frame #12 {
        n237 = VISA Flush I/O Buffer(VISA resource name=w786, error in (no error)=w787) -> (VISA resource name out=w785:refnum<visa-resource-name>, error out=w784:errorcluster)  [unwired: 1 in]
        n238 = VISA Close(VISA resource name=w785, error in (no error)=w784) -> (error out=→"Ion Gauge Controller":errorcluster)
      }
    }
    n239 = flat-sequence {
      tunnel: w245 -> [w254]
      tunnel: w244 -> [w253]
      tunnel: [w252] -> w224
      tunnel: [w251] -> w223
      tunnel: [w249] -> w222
      tunnel: w224 -> [w273]
      tunnel: w223 -> [w274]
      tunnel: [w267] -> w221
      tunnel: [w266] -> w220
      tunnel: [w265] -> w219
      tunnel: w222 -> [w265]
      tunnel: w221 -> [w290]
      tunnel: w220 -> [w289]
      tunnel: [w287] -> w218
      tunnel: [w286] -> w217
      tunnel: [w285] -> w216
      tunnel: w219 -> [w285]
      tunnel: w218 -> [w313]
      tunnel: w217 -> [w312]
      tunnel: [w311] -> w215
      tunnel: [w310] -> w214
      tunnel: [w309] -> w213
      tunnel: w216 -> [w309]
      tunnel: [w301] -> w212
      tunnel: w215 -> [w336]
      tunnel: w214 -> [w335]
      tunnel: [w334] -> w211
      tunnel: [w333] -> w210
      tunnel: [w332] -> w209
      tunnel: w213 -> [w332]
      tunnel: w212 -> [w328]
      tunnel: [w328] -> w208
      tunnel: w211 -> [w354]
      tunnel: w210 -> [w355]
      tunnel: [w353] -> w207
      tunnel: [w352] -> w206
      tunnel: [w351] -> w205
      tunnel: w209 -> [w351]
      tunnel: [w348] -> w204
      tunnel: w208 -> [w347]
      tunnel: [w347] -> w203
      tunnel: w207 -> [w375]
      tunnel: w206 -> [w374]
      tunnel: [w373] -> w202
      tunnel: w205 -> [w373]
      tunnel: [w372] -> w201
      tunnel: [w371] -> w200
      tunnel: [w370] -> w199
      tunnel: w204 -> [w370]
      tunnel: w203 -> [w369]
      tunnel: [w369] -> w198
      tunnel: w202 -> [w398]
      tunnel: [w396] -> w197
      tunnel: w201 -> [w396]
      tunnel: w200 -> [w395]
      tunnel: [w395] -> w196
      tunnel: w199 -> [w387]
      tunnel: [w393] -> w195
      tunnel: w198 -> [w392]
      tunnel: [w392] -> w194
      tunnel: [w386] -> w130
      tunnel: w197 -> [w406]
      tunnel: w196 -> [w405]
      tunnel: w195 -> [w400]
      tunnel: w194 -> [w403]
      tunnel: [w400] -> w125
      tunnel: w125 -> [w446]
      frame #0 {
        n240 = Concatenate Strings("#01VER", "\r") -> (w262:string)
        n241 = Wait (ms)(milliseconds to wait=50) -> ()  [unwired: 1 out]
        n242 = VISA Write(VISA resource name=w254, write buffer=w262, error in (no error)=w253) -> (VISA resource name out=w258:refnum<visa-resource-name>, error out=w257:errorcluster)  [unwired: 1 out]
        n243 = VISA Read(VISA resource name=w258, byte count=13, error in (no error)=w257) -> (VISA resource name out=w252:refnum<visa-resource-name>, read buffer=w255:string, error out=w251:errorcluster)  [unwired: 1 out]
        n244 = Concatenate Strings(" 1770-107", "\r") -> (w246:string)
        n245 = Search/Split String(string=w255, search string/char (-)=" ", offset (0)=3) -> (match + rest of string=w250:string)  [unwired: 2 out]
        "Software Version" <- w250
        n246 = Equal?(x=w246, y=w250) -> (x = y?=w249:bool)
      }
      frame #1 {
        n247 = Concatenate Strings("#01RS", "\r") -> (w277:string)
        n248 = Wait (ms)(milliseconds to wait=50) -> ()  [unwired: 1 out]
        n249 = VISA Write(VISA resource name=w273, write buffer=w277, error in (no error)=w274) -> (VISA resource name out=w281:refnum<visa-resource-name>, error out=w282:errorcluster)  [unwired: 1 out]
        n250 = VISA Read(VISA resource name=w281, byte count=13, error in (no error)=w282) -> (VISA resource name out=w267:refnum<visa-resource-name>, read buffer=w284:string, error out=w266:errorcluster)  [unwired: 1 out]
        n251 = Search/Split String(string=w284, search string/char (-)=" ", offset (0)=3) -> (match + rest of string=w270:string)  [unwired: 2 out]
        n252 = Search/Split String(string=w270, search string/char (-)=" ", offset (0)=3) -> (substring before match=→"IG Code\nIG code":string, match + rest of string=→"IG Status":string)  [unwired: 1 out]
      }
      frame #2 {
        n253 = Concatenate Strings("#01SES", "\r") -> (w293:string)
        n254 = Wait (ms)(milliseconds to wait=50) -> ()  [unwired: 1 out]
        n255 = VISA Write(VISA resource name=w290, write buffer=w293, error in (no error)=w289) -> (VISA resource name out=w297:refnum<visa-resource-name>, error out=w298:errorcluster)  [unwired: 1 out]
        n256 = VISA Read(VISA resource name=w297, byte count=13, error in (no error)=w298) -> (VISA resource name out=w287:refnum<visa-resource-name>, read buffer=w300:string, error out=w286:errorcluster)  [unwired: 1 out]
        n257 = Search/Split String(string=w300, search string/char (-)=" ", offset (0)=3) -> (match + rest of string=→"Emission Current Status":string)  [unwired: 2 out]
      }
      frame #3 {
        n258 = Concatenate Strings("#01IGS", "\r") -> (w316:string)
        n259 = Wait (ms)(milliseconds to wait=50) -> ()  [unwired: 1 out]
        n260 = VISA Write(VISA resource name=w313, write buffer=w316, error in (no error)=w312) -> (VISA resource name out=w320:refnum<visa-resource-name>, error out=w321:errorcluster)  [unwired: 1 out]
        n261 = VISA Read(VISA resource name=w320, byte count=13, error in (no error)=w321) -> (VISA resource name out=w311:refnum<visa-resource-name>, read buffer=w323:string, error out=w310:errorcluster)  [unwired: 1 out]
        n262 = Search/Split String(string=w323, search string/char (-)="IG ", offset (0)=3) -> (match + rest of string=w302:string)  [unwired: 2 out]
        "IG Filament Status" <- w302
        n263 = Search/Split String(string=w302, search string/char (-)="O", offset (0)=3) -> (match + rest of string=w303:string)  [unwired: 2 out]
        n264 = Concatenate Strings("OFF", "\r") -> (w304:string)
        n265 = Equal?(x=w304, y=w303) -> (x = y?=w301:bool)
        n266 = case shown="False" w301 {
          frame False {
            w324 = TRUE
            n267 = local write "Apagado"(FALSE ("Apagado")) -> ()
            "Activo" <- w324
            "ActivoIG" <- w324
          }
          frame True {
            w327 = FALSE
            n268 = local write "ActivoIG"(w327) -> ()
            n269 = local write "Activo"(w327) -> ()
            "Apagado" <- TRUE ("Apagado")
          }
        }
      }
      frame #4 {
        n270 = Concatenate Strings("#01RDCG1", "\r") -> (w344:string)
        n271 = Wait (ms)(milliseconds to wait=50) -> ()  [unwired: 1 out]
        n272 = VISA Write(VISA resource name=w336, write buffer=w344, error in (no error)=w335) -> (VISA resource name out=w340:refnum<visa-resource-name>, error out=w339:errorcluster)  [unwired: 1 out]
        n273 = VISA Read(VISA resource name=w340, byte count=13, error in (no error)=w339) -> (VISA resource name out=w333:refnum<visa-resource-name>, read buffer=w337:string, error out=w334:errorcluster)  [unwired: 1 out]
        n274 = Search/Split String(string=w337, search string/char (-)=" ", offset (0)=3) -> (match + rest of string=w330:string)  [unwired: 2 out]
        "CG1 [TORR]" <- w330
        n275 = Fract/Exp String To Number(use system decimal point (T)=TRUE, string=w330) -> (number=→"CG1L" →"CG1":dbl)  [unwired: 2 in, 1 out]
      }
      frame #5 {
        n276 = Concatenate Strings("#01RDCG2", "\r") -> (w358:string)
        n277 = Wait (ms)(milliseconds to wait=50) -> ()  [unwired: 1 out]
        n278 = VISA Write(VISA resource name=w355, write buffer=w358, error in (no error)=w354) -> (VISA resource name out=w362:refnum<visa-resource-name>, error out=w363:errorcluster)  [unwired: 1 out]
        n279 = VISA Read(VISA resource name=w362, byte count=13, error in (no error)=w363) -> (VISA resource name out=w353:refnum<visa-resource-name>, read buffer=w365:string, error out=w352:errorcluster)  [unwired: 1 out]
        n280 = Search/Split String(string=w365, search string/char (-)=" ", offset (0)=3) -> (match + rest of string=w349:string)  [unwired: 2 out]
        "CG2 [TORR]" <- w349
        n281 = Fract/Exp String To Number(use system decimal point (T)=TRUE, string=w349) -> (number=w348:dbl)  [unwired: 2 in, 1 out]
        "CG2L" <- w348
        "CG2" <- w348
      }
      frame #6 {
        n282 = Concatenate Strings("#01RD", "\r") -> (w378:string)
        n283 = Wait (ms)(milliseconds to wait=50) -> ()  [unwired: 1 out]
        n284 = VISA Write(VISA resource name=w375, write buffer=w378, error in (no error)=w374) -> (VISA resource name out=w382:refnum<visa-resource-name>, error out=w383:errorcluster)  [unwired: 1 out]
        n285 = VISA Read(VISA resource name=w382, byte count=13, error in (no error)=w383) -> (VISA resource name out=w372:refnum<visa-resource-name>, read buffer=w385:string, error out=w371:errorcluster)  [unwired: 1 out]
        n286 = Search/Split String(string=w385, search string/char (-)=" ", offset (0)=3) -> (match + rest of string=w367:string)  [unwired: 2 out]
        "IG [TORR]" <- w367
        n287 = Fract/Exp String To Number(use system decimal point (T)=TRUE, string=w367) -> (number=→"IG3" →"IG" →"IG1" →"IG2":dbl)  [unwired: 2 in, 1 out]
      }
      frame #7 {
        n288 = And(x=TRUE, y=w398) -> (x .and. y?=→"IG_Online":bool)
        n289 = Greater Or Equal?(x=w387, y=740.0) -> (x >= y?=w390:bool)
        n290 = Greater Or Equal?(x=8.0 ("y"), y=w387) -> (x >= y?=w386:bool)
        "TP AV/NAV" <- w386
        n291 = Greater Or Equal?(x=0.001, y=w387) -> (x >= y?=w393:bool)
        n292 = Not(x=w390) -> (.not. x?=→"VAC/ATM":bool)
      }
      frame #8 {
        n293 = And(x="Ion Gauge", y=w400) -> (x .and. y?=w404:bool)
        n294 = case shown="False" w404 {
          tunnel: w406 -> [w410 w428]
          tunnel: w405 -> [w409 w427]
          tunnel: w403 -> [w408 w426]
          tunnel: [w407 w425] -> w402
          frame False {
            n295 = Wait (ms)(milliseconds to wait=50) -> ()  [unwired: 1 out]
            n296 = case shown="True" w408 {
              tunnel: w410 -> [w420 w424]
              tunnel: w409 -> [w419 w423]
              tunnel: [w412 w421] -> w407
              frame False {
                n297 = Concatenate Strings("#01IG0", "\r") -> (w416:string)
                n298 = Wait (ms)(milliseconds to wait=10000) -> ()  [unwired: 1 out]
                n299 = VISA Write(VISA resource name=w420, write buffer=w416, error in (no error)=w419) -> (VISA resource name out=w414:refnum<visa-resource-name>, error out=w413:errorcluster)  [unwired: 1 out]
                n300 = VISA Close(VISA resource name=w414, error in (no error)=w413) -> (error out=w412:errorcluster)
              }
              frame True {
                n301 = VISA Close(VISA resource name=w424, error in (no error)=w423) -> (error out=w421:errorcluster)
                n302 = Wait (ms)(milliseconds to wait=50) -> ()  [unwired: 1 out]
              }
            }
          }
          frame True {
            n303 = Wait (ms)(milliseconds to wait=50) -> ()  [unwired: 1 out]
            n304 = case shown="True" w426 {
              tunnel: w428 -> [w432 w439]
              tunnel: w427 -> [w431 w438]
              tunnel: [w430 w434] -> w425
              frame False {
                n305 = Wait (ms)(milliseconds to wait=50) -> ()  [unwired: 1 out]
                n306 = VISA Close(VISA resource name=w432, error in (no error)=w431) -> (error out=w430:errorcluster)
              }
              frame True {
                n307 = Concatenate Strings("#01IG1", "\r") -> (w441:string)
                n308 = Wait (ms)(milliseconds to wait=10000) -> ()  [unwired: 1 out]
                n309 = VISA Write(VISA resource name=w439, write buffer=w441, error in (no error)=w438) -> (VISA resource name out=w437:refnum<visa-resource-name>, error out=w436:errorcluster)  [unwired: 1 out]
                n310 = VISA Close(VISA resource name=w437, error in (no error)=w436) -> (error out=w434:errorcluster)
              }
            }
          }
        }
        "Vacuum Controller" <- w402
        "IG AV/NAV" <- w400
        "IG AV/NAV 2" <- w400
      }
      frame #9 {
        n311 = case shown="False" w446 {
          frame False {
            n312 = local write "Ion Gauge"(FALSE ("Ion Gauge")) -> ()
          }
          frame True {
          }
        }
        n313 = Or(x="System ON", y="System OFF") -> (x .or. y?=w445:bool)
        n314 = case shown="True" w445 {
          tunnel: "System ON" -> [_ w449]
          tunnel: "System OFF" -> [_ w447]
          frame False {
          }
          frame True {
            n315 = flat-sequence {
              tunnel: w449 -> [w451]
              tunnel: [w450] -> w448
              tunnel: w447 -> [w450]
              tunnel: w448 -> [w454]
              frame #0 {
                n316 = case shown="False" w451 {
                  frame False {
                  }
                  frame True {
                    w452 = TRUE ("Turbo Pump")
                    n317 = local write "Turbo Pump"(w452) -> ()
                    n318 = local write "Backing Pump"(w452) -> ()
                    n319 = local write "System OFF"(FALSE ("System OFF")) -> ()
                  }
                }
              }
              frame #1 {
                n320 = case shown="True" w454 {
                  frame False {
                  }
                  frame True {
                    w455 = FALSE ("Turbo Pump")
                    n321 = local write "Turbo Pump"(w455) -> ()
                    n322 = local write "Backing Pump"(w455) -> ()
                    n323 = local write "System ON"(FALSE ("System ON")) -> ()
                  }
                }
              }
            }
          }
        }
      }
    }
  }
